vi "Close.vi"(8 "error in (no error)":errorcluster, 11 "LiFingerprint in":refnum<class "LiFingerprint.lvclass">) -> (0 "error out":errorcluster)   [LabVIEW 2020, in "LiFingerprint.lvclass"]
uses:
  LiFingerprint.lvclass
  LiFingerprint.lvclass/LiFingerprint.ctl
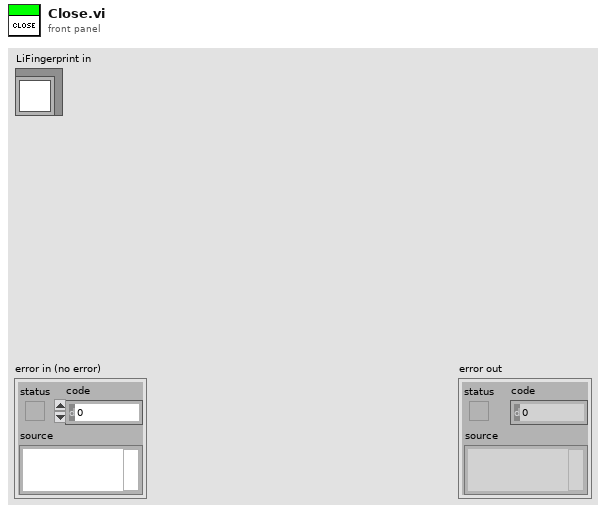
[diagram p1: front panel]
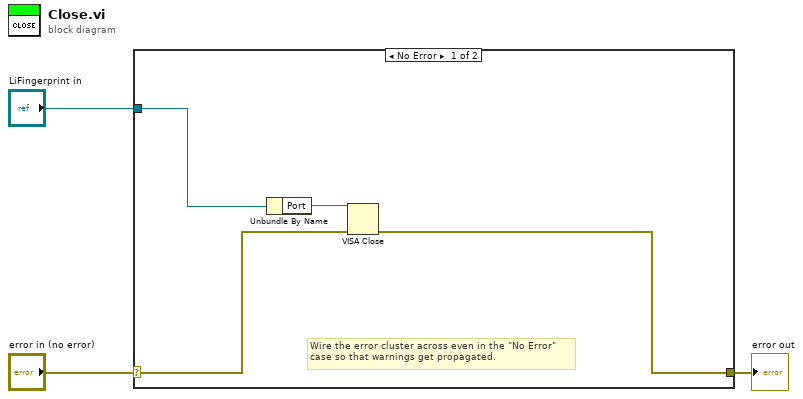
[diagram p0: block diagram]
diagram:
  n1 = case shown="No Error" "error in (no error)" {
    selector: "error in (no error)" -> [w5 w8]
    tunnel: [w4 w8] -> w2
    tunnel: "LiFingerprint in" -> [w7 _]
    frame No Error {
      # "Wire the error cluster across even in the \"No Error\"\ncase so that warnings get propagated."
      n2 = Unbundle By Name(w7) -> ("Port"=w6:refnum<visa-resource-name>)
      n3 = VISA Close(VISA resource name=w6, error in (no error)=w5) -> (error out=w4:errorcluster)
    }
    frame Error {
    }
  }
  "error out" <- w2
